vi "Calcul itératif.vi"(10 "Température capteur 1-2-3-4-Ambiant":dbl[](array[numeric]), 11 "Position des capteurs":dbl[][](array[numeric])) -> ()   [LabVIEW 2018]
panel:
  in  "DiffR":dbl
  in  "T max":dbl
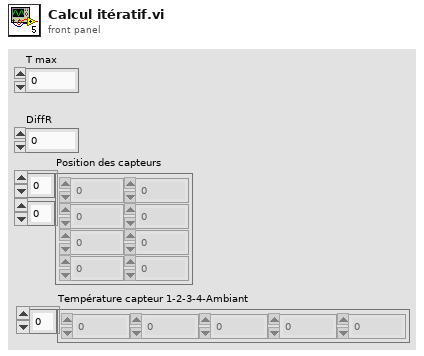
[diagram p1: front panel]
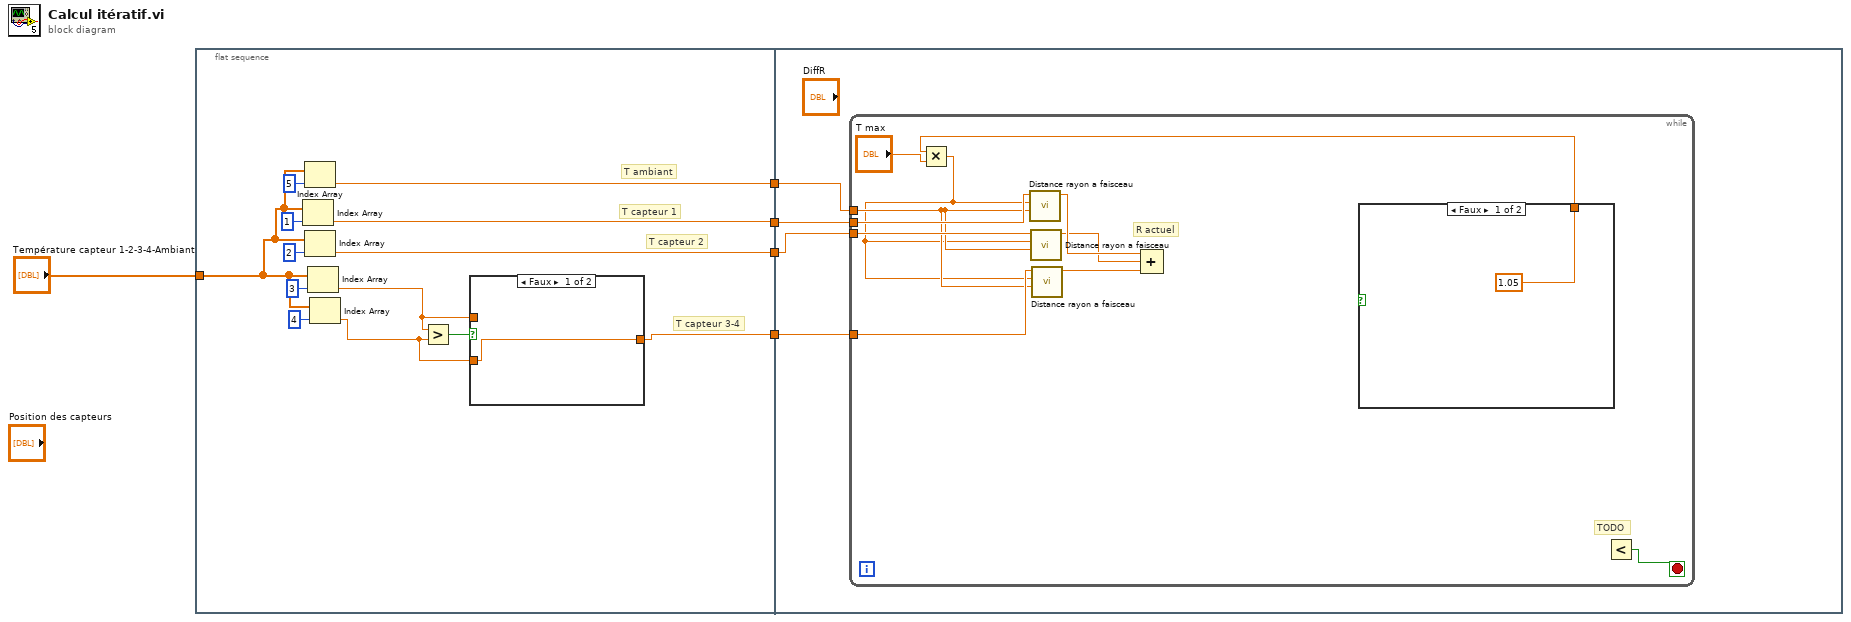
[diagram p0: block diagram]
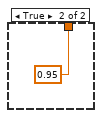
[diagram p3: hidden frame]
diagram:
  n1 = flat-sequence {
    tunnel: "Température capteur 1-2-3-4-Ambiant" -> [w8]
    tunnel: [w14] -> w4
    tunnel: [w10] -> w3
    tunnel: [w9] -> w2
    tunnel: [w6] -> w1
    tunnel: w4 -> [w21]
    tunnel: w3 -> [w24]
    tunnel: w2 -> [w22]
    tunnel: w1 -> [w23]
    frame #0 {
      # "T capteur 3-4"
      # "T capteur 2"
      # "T capteur 1"
      # "T ambiant"
      n2 = Index Array(array=w8, index=1 ("indice")) -> (element=w10:dbl)
      n3 = Index Array(array=w8, index=5 ("indice")) -> (element=w6:dbl)
      n4 = Index Array(array=w8, index=2 ("indice")) -> (element=w9:dbl)
      n5 = Index Array(array=w8, index=3 ("indice")) -> (element=w15:dbl)
      n6 = Index Array(array=w8, index=4 ("indice")) -> (element=w13:dbl)
      n7 = Greater?(x=w15, y=w13) -> (0:w16:bool)
      n8 = case shown="Faux" w16 {
        tunnel: [w19 w20] -> w14
        tunnel: w15 -> [_ w20]
        tunnel: w13 -> [w19 _]
        frame False {
        }
        frame True {
        }
      }
    }
    frame #1 {
      n9 = while {
        tunnel: w24 -> [w34]
        tunnel: w23 -> [w31]
        tunnel: w22 -> [w33]
        tunnel: w21 -> [w32]
        stop <- w35 stop-if-true
        # "R actuel"
        # "TODO"
        n10 = case shown="Faux" {
          selector: _ -> [_ _]
          tunnel: [1.05 0.95] -> w25
          frame False {
          }
          frame True {
          }
        }
        n11 = Multiply(x=w25, y="T max") -> (x*y=w26:dbl)
        n12 = call "Distance rayon a faisceau.vi"("T ambiant"=w31, "T max"=w26, "T capteur"=w34) -> ("Rayon"=w30:dbl)  [unwired: 8 in]
        n13 = call "Distance rayon a faisceau.vi"("T ambiant"=w31, "T max"=w26, "T capteur"=w33) -> ("Rayon"=w29:dbl)  [unwired: 8 in]
        n14 = call "Distance rayon a faisceau.vi"("T ambiant"=w31, "T max"=w26, "T capteur"=w32) -> ("Rayon"=w28:dbl)  [unwired: 8 in]
        n15 = Compound Arithmetic op=ADD(w30, w29, w28) -> ()  [unwired: 1 out]
        n16 = Less?() -> (x < y?=w35:bool)  [unwired: 2 in]
      }
    }
  }
